vi "Module Top Level.vi"(8 "error in (no error)":errorcluster) -> (0 "error out":errorcluster)   [LabVIEW 2018, in "Controller (Host).lvlib"]
doc: "This is the top level VI for this module. It uses a queue for communications and is stopped using a user event. The general architecture is similar to a simple queued message handler.\n\nThis module controls the host computer logic, specifically the following:\nSplash screen deployment for user selections (APU selection, Operation selection)\nUser Interface visual deployment during operation"
uses:
  Controller (Host).lvlib
  Private Controls/Controller (Host) Data.ctl
  Private Controls/State.ctl
  Top Level/Shared Controls/APU Setup File.ctl
  Public Controls/Test Information.ctl
  Public VIs/PreorPostSB.ctl
  Public Controls/APU Select.ctl
  Top Level/Shared Controls/Calculated Data.ctl
  Private Controls/Module Data.ctl
  Private Controls/Module Action.ctl
  Top Level/Shared Controls/All Data Cluster.ctl
  Top Level/Shared Controls/Acq Data.ctl
  Globals/Host Globals.vi
  Error Handler/Error Handler.lvlib
  File IO/File IO.lvlib
  Testing UI 1/Testing UI 1.lvlib
  Testing UI 3/Testing UI 3.lvlib
  Testing UI 2/Testing UI 2.lvlib
  Fuel Farm/Fuel Farm.lvlib
panel:
  # "CONTROLLER"
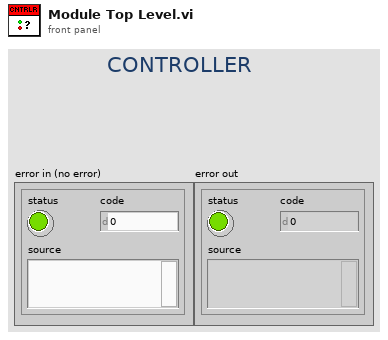
[diagram p1: front panel]
types:
  T1 = typedef "Controller (Host).lvlib/Controller (Host) Data.ctl" = cluster{"State":T2, "2D User Info":string[][], "APU Setup File":T3, "Test Information":T4, "ChannelTags":string[], "Live_Min_Max_Dev":dbl[][], "CalChannels":string[], "Slopes":dbl[], "Offsets":dbl[], "Calculated Values":T7, "ThresholdChannels":string[], "ThresholdRPM":dbl[], "ThresholdMin":bool[], "ThresholdValue":dbl[], "HeavyCCM":dbl[][], "LightCCM":dbl[][], "FuelFarm":bool}
  T2 = typedef "Controller (Host).lvlib/State.ctl" = enum16{"APU Select", "Operation Select", "SubTests Select", "Calibration", "Testing", "Exit"}
  T3 = typedef "APU Setup File.ctl" = cluster{"Sensor Info":string[][], "Variables":string[][], "CMM Table 106":string[][], "CMM Table 106B ":string[][], "Accel Config":string[][], "Report Sheet 1":string[][], "Report Sheet 2":string[][], "Report Sheet 3":string[][]}
  T4 = typedef "Controller (Host).lvlib/Test Information.ctl" = cluster{"APU Part Number:":string, "Model:":string, "Serial Number:":string, "Customer:":string, "Work Order:":string, "Pre or Post SB":T5, "Run Count":i32, "APU Selected":T6}
  T5 = typedef "Controller (Host).lvlib/PreorPostSB.ctl" = string
  T6 = typedef "Controller (Host).lvlib/APU Select.ctl" = string
  T7 = typedef "Calculated Data.ctl" = cluster{"C.00":dbl, "C.01":dbl, "C.02":dbl, "C.03":dbl, "C.04":dbl, "C.05":dbl, "C.06":dbl, "C.07":dbl, "C.08":dbl, "C.09":dbl, "C.10":dbl, "C.11":dbl, "C.12":dbl, "C.13":dbl, "C.14":dbl, "C.15":dbl, "C.16":dbl, "C.17":dbl, "C.18":dbl, "C.19":dbl, "C.20":dbl, "C.21":dbl, "C.22":dbl, "C.23":dbl, "C.24":dbl, "C.25":dbl, "C.26":dbl, "C.27":dbl, "C.28":dbl, "C.29":dbl, "C.30":dbl, "C.31":dbl, "C.32":dbl, "C.33":dbl, "C.34":dbl, "C.35":dbl, "C.36":dbl, "C.37":dbl, "C.38":dbl, "C.39":dbl, "C.40":dbl, "C.41":dbl, "C.42":dbl, "C.43":dbl, "C.44":dbl, "C.45":dbl, "C.46":dbl, "C.47":dbl, "C.48":dbl, "C.49":dbl, "C.50":dbl, "C.51":dbl, "C.52":dbl, "C.53":dbl, "C.54":dbl, "C.55":dbl, "C.56":dbl, "C.57":dbl, "C.58":dbl, "C.59":dbl, "C.60":dbl, "C.61":dbl, "C.62":dbl}
  T8 = typedef "All Data Cluster.ctl" = cluster{"AI":T9, "Accel Data":cluster{"Accel RMS(in/sec2)":dbl[], "Accel Peak(in/sec2)":dbl[], "Velocity RMS(in/sec)":dbl[], "Velocity Peak(in/sec)":dbl[]}, "Temps":cluster{"01-00-9213":dbl[], "01-01-9213":dbl[], "01-02-9213":dbl[]}, "00-03-9402(RPM)":dbl[], "02-04-9871":dbl[], "ARINC":sgl[]}
  T9 = typedef "Acq Data.ctl" = cluster{"00-00-9220":dbl[], "00-01-9220":dbl[], "02-02-9219":dbl[], "02-03-9227":dbl[], "02-05-9205":dbl[]}
  T10 = typedef "Controller (Host).lvlib/Module Data.ctl" = cluster{"Data":variant, "Action":T11}
  T11 = typedef "Controller (Host).lvlib/Module Action.ctl" = enum8{"Timeout", "New Data", "Value to Monitor", "Init", "Reset Dev_Min_Max", "Error", "Exit", "Prompt Test Info", "Update Test Info", "Prompt Variable Info", "Load APU Setup Data"}
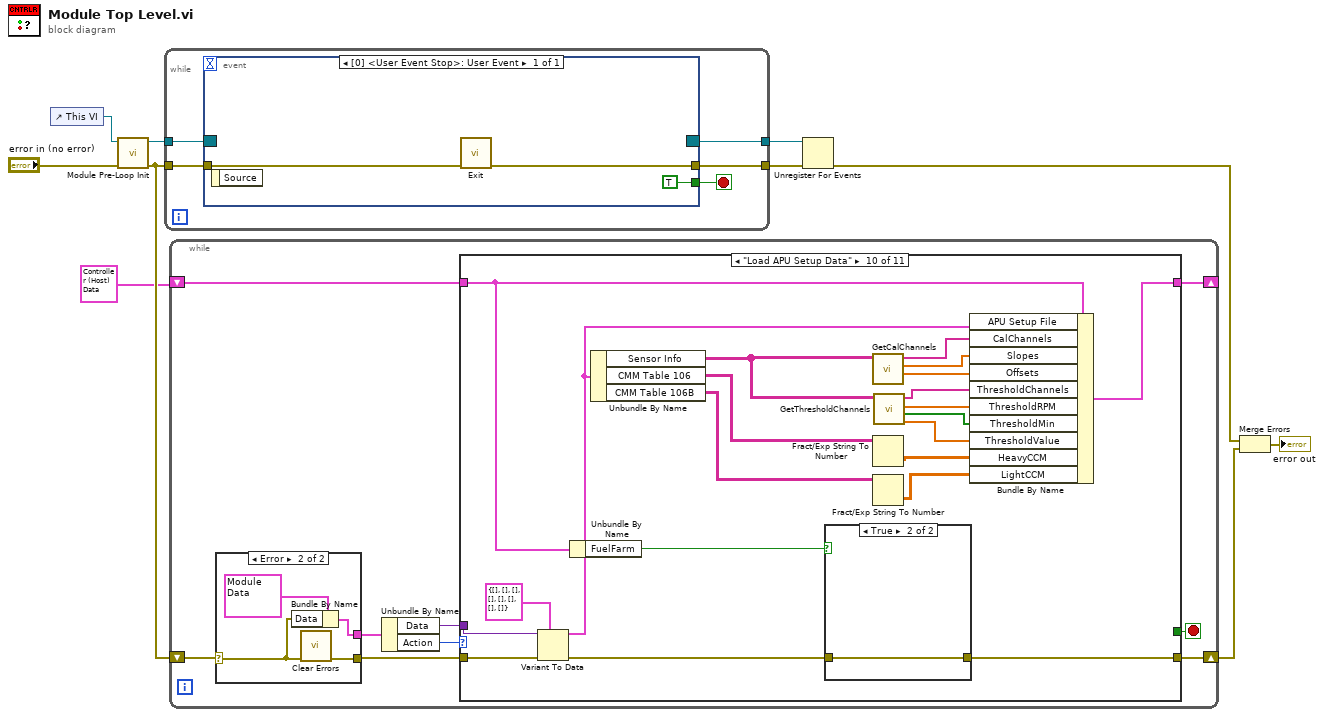
[diagram p0: block diagram]
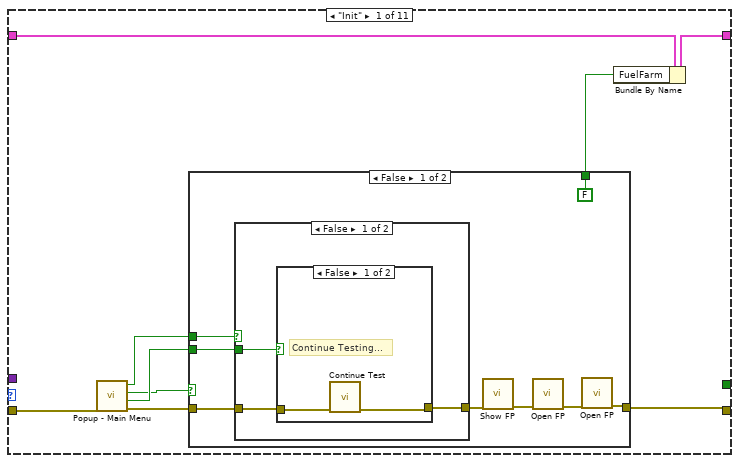
[diagram p2: hidden frame]
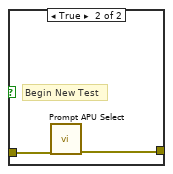
[diagram p3: hidden frame]
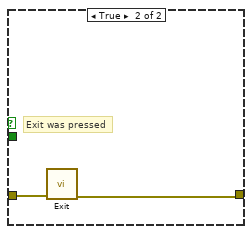
[diagram p4: hidden frame]
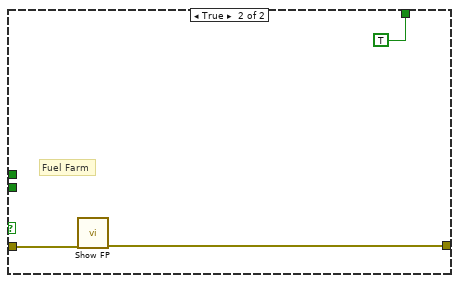
[diagram p5: hidden frame]
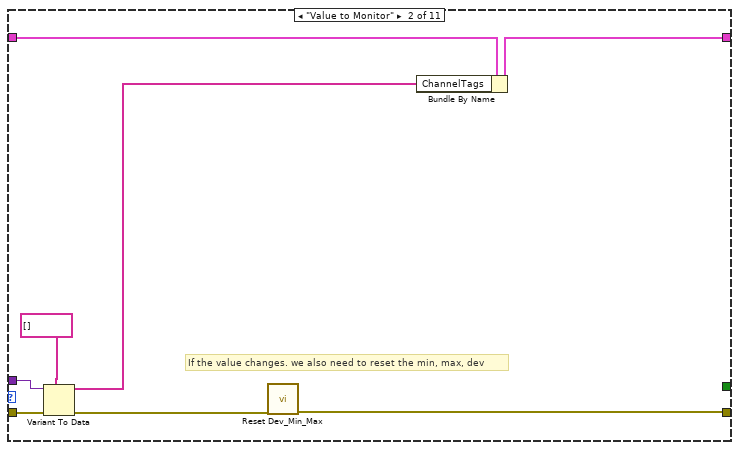
[diagram p6: hidden frame]
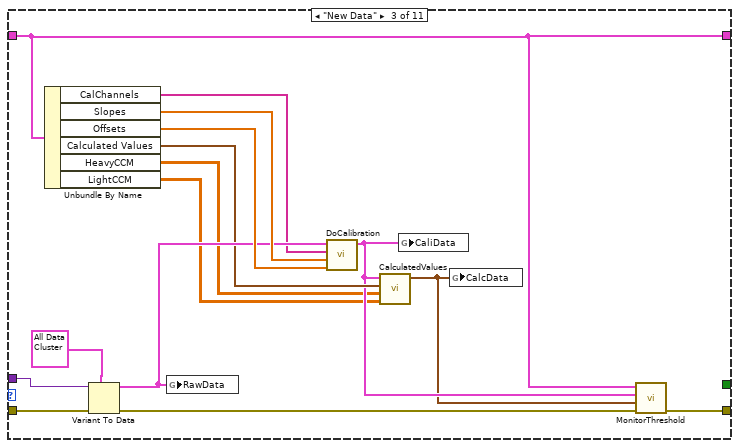
[diagram p7: hidden frame]
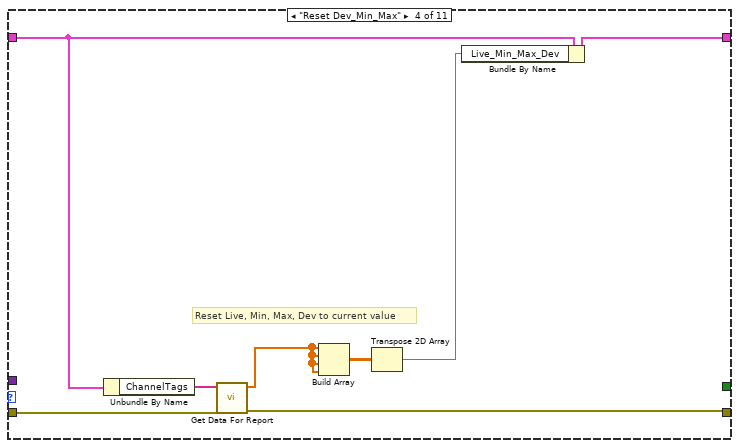
[diagram p8: hidden frame]
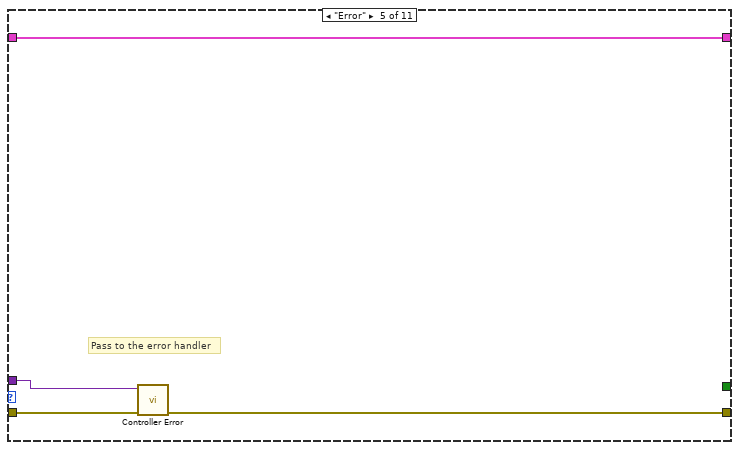
[diagram p9: hidden frame]
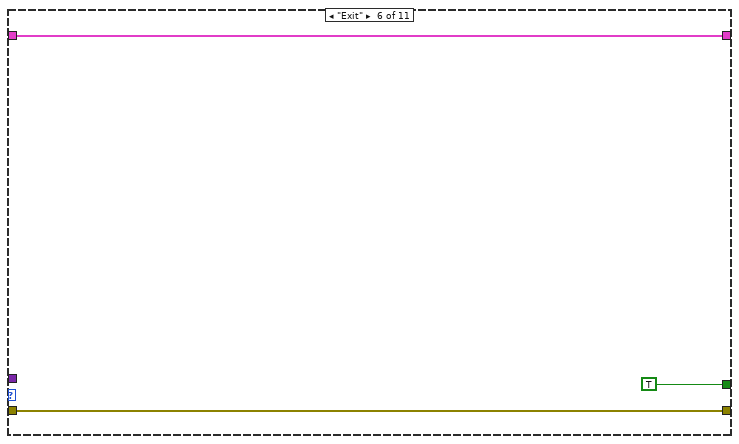
[diagram p10: hidden frame]
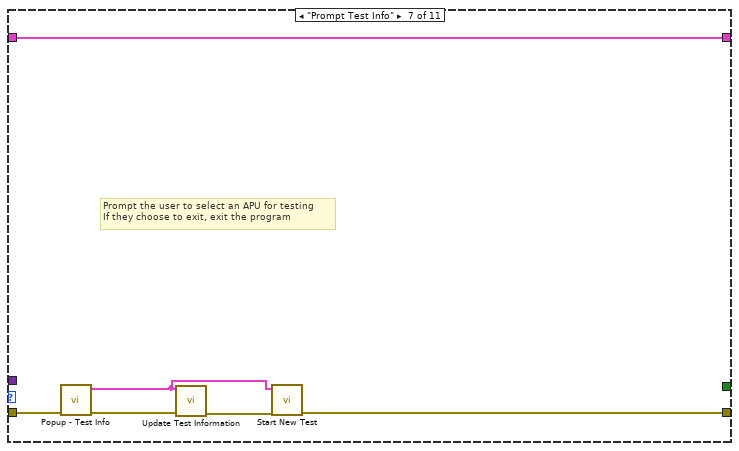
[diagram p11: hidden frame]
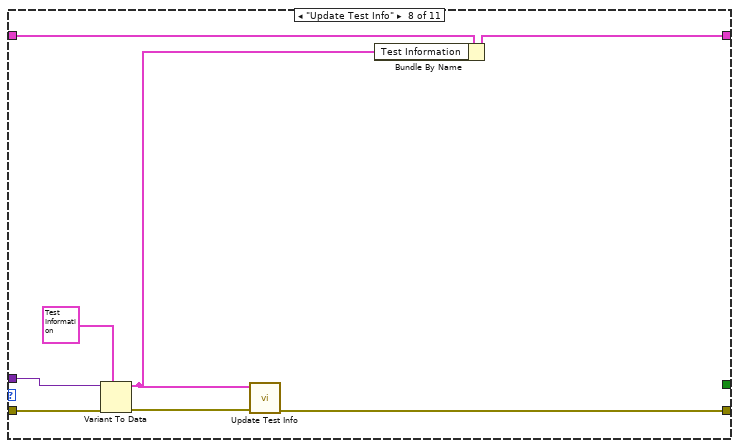
[diagram p12: hidden frame]
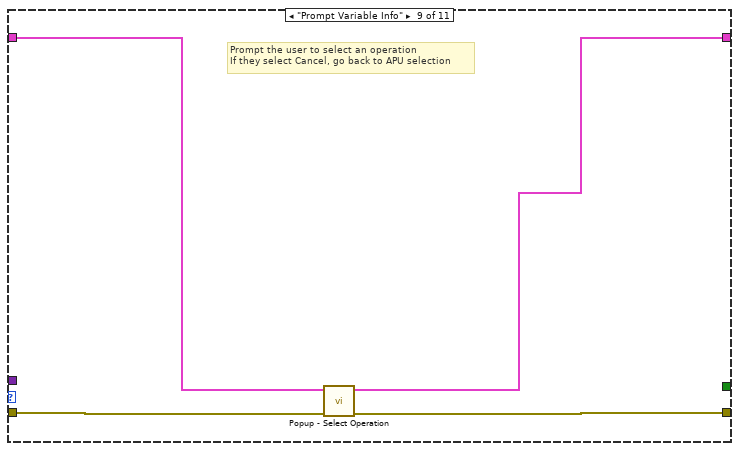
[diagram p13: hidden frame]
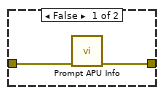
[diagram p14: hidden frame]
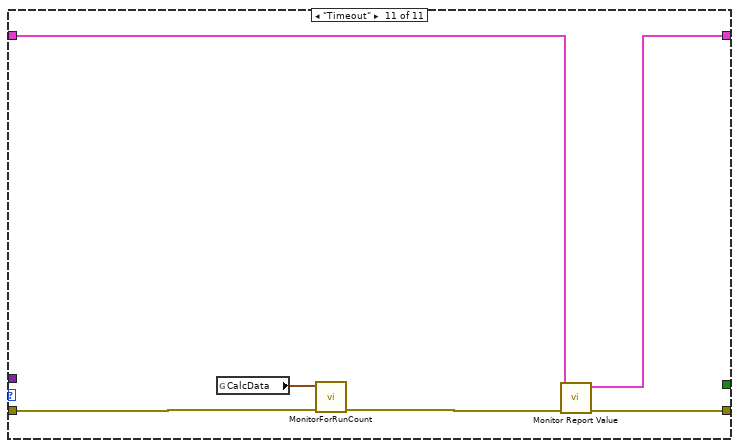
[diagram p15: hidden frame]
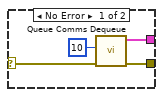
[diagram p16: hidden frame]
diagram:
  n1 = control-ref of="This VI"() -> (w10:refnum<vi>)
  n2 = call "Module Pre-Loop Init.vi"("error in (no error)"="error in (no error)", "Top Level VI Ref in"=w10) -> ("error out"=w2:errorcluster, "User Event Stop Ref"=w8:refnum<event-registration>)  [unwired: 8 in]
  n3 = while {
    tunnel: w8 -> [w15]
    tunnel: [w14] -> w6
    tunnel: w2 -> [w13]
    tunnel: [w11] -> w7
    stop <- w12 stop-if-true
    n4 = event shown="[0] <User Event Stop>: User Event" {
      selector: w15 -> [_]
      dyn-events: [_] -> w11
      timeout: _ -> [_]
      tunnel: [w16] -> w14
      tunnel: w13 -> [w17]
      tunnel: [TRUE] -> w12
      event User Event {
        n5 = event-data() -> ()  [unwired: 1 in, 1 out]
        n6 = call "Exit.vi"("error in"=w17) -> ("error out"=w16:errorcluster)  [unwired: 10 in]
      }
    }
  }
  n7 = while {
    shift-right: [w23] -> w5
    shift-left: w2 -> [w22]
    shift-right: [w21] -> _
    shift-left: T1 {"State"=enum."APU Select", "2D User Info"=[], "APU Setup File"={"Sensor Info"=[], "Variables"=[], "CMM Table 106"=[], "CMM Table 106B "=[], "Accel Config"=[], "Report Sheet 1"=[], "Report Sheet 2"=[], "Report Sheet 3"=[]}, "Test Information"={"APU Part Number:"="", "Model:"="", "Serial Number:"="", "Customer:"="", "Work Order:"="", "Pre or Post SB"="", "Run Count"=0, "APU Selected"="<Select>"}, "ChannelTags"=[], "Live_Min_Max_Dev"=[], "CalChannels"=[], "Slopes"=[], "Offsets"=[], "Calculated Values"={"C.00"=0.0, "C.01"=0.0, "C.02"=0.0, "C.03"=0.0, "C.04"=0.0, "C.05"=0.0, "C.06"=0.0, "C.07"=0.0, "C.08"=0.0, "C.09"=0.0, "C.10"=0.0, "C.11"=0.0, "C.12"=0.0, "C.13"=0.0, "C.14"=0.0, "C.15"=0.0, "C.16"=0.0, "C.17"=0.0, "C.18"=0.0, "C.19"=0.0, "C.20"=0.0, "C.21"=0.0, "C.22"=0.0, "C.23"=0.0, "C.24"=0.0, "C.25"=0.0, "C.26"=0.0, "C.27"=0.0, "C.28"=0.0, "C.29"=0.0, "C.30"=0.0, "C.31"=0.0, "C.32"=0.0, "C.33"=0.0, "C.34"=0.0, "C.35"=0.0, "C.36"=0.0, "C.37"=0.0, "C.38"=0.0, "C.39"=0.0, "C.40"=0.0, "C.41"=0.0, "C.42"=0.0, "C.43"=0.0, "C.44"=0.0, "C.45"=0.0, "C.46"=0.0, "C.47"=0.0, "C.48"=0.0, "C.49"=0.0, "C.50"=0.0, "C.51"=0.0, "C.52"=0.0, "C.53"=0.0, "C.54"=0.0, "C.55"=0.0, "C.56"=0.0, "C.57"=0.0, "C.58"=0.0, "C.59"=0.0, "C.60"=0.0, "C.61"=0.0, "C.62"=0.0}, "ThresholdChannels"=[], "ThresholdRPM"=[], "ThresholdMin"=[], "ThresholdValue"=[], "HeavyCCM"=[], "LightCCM"=[], "FuelFarm"=FALSE} -> [w20]
    stop <- w24 stop-if-true
    n8 = case shown="Error" w22 {
      selector: w22 -> [w145 w148]
      tunnel: [w146 w149] -> w27
      tunnel: [w144 w147] -> w25
      frame No Error {
        n9 = call "Queue Comms Dequeue.vi"("error in (no error)"=w145, "timeout in ms (-1)"=10) -> ("error out"=w144:errorcluster, "element"=w146:T10)  [unwired: 8 in]
      }
      frame Error {
        n10 = Bundle By Name(cluster=T10 {"Data"=variant, "Action"=enum."Error"} ("element"), "Data"=w148) -> (w149:T10)
        n11 = call <vilib>:"Clear Errors.vi"("error in (no error)"=w148) -> ("error out"=w147:errorcluster)  [unwired: 5 in, 1 out]
      }
    }
    n12 = Unbundle By Name(w27) -> ("Data"=w26:variant, "Action"=w19:T11)
    n13 = case shown="\"Load APU Setup Data\"" w19 {
      tunnel: w26 -> [_ w61 w78 _ w89 _ _ w106 _ w133 _]
      tunnel: w25 -> [w35 w63 w79 w87 w91 w93 w99 w107 w112 w132 w142]
      tunnel: [w36 w57 w68 w83 w90 w93 w96 w102 w111 w129 w140] -> w23
      tunnel: [_ _ _ _ _ TRUE _ _ _ _ _] -> w24
      tunnel: [w29 w60 w67 w84 w88 w92 w100 w104 w110 w127 w139] -> w21
      tunnel: w20 -> [w30 w64 w67 w86 w88 w92 w100 w108 w109 w114 w138]
      frame "Init" {
        n14 = call "Popup - Main Menu.vi"("error in"=w35) -> ("error out"=w34:errorcluster, "IsNewTest"=w33:bool, "FuelFarm"=w31:bool, "Exit"=w32:bool)  [unwired: 7 in]
        n15 = case shown="False" w31 {
          tunnel: [w38 w55] -> w36
          tunnel: w34 -> [w44 w56]
          tunnel: w33 -> [w43 _]
          tunnel: w32 -> [w42 _]
          tunnel: [FALSE TRUE] -> w28
          frame False {
            n16 = case shown="False" w42 {
              tunnel: [w47 w52] -> w41
              tunnel: w44 -> [w46 w53]
              tunnel: w43 -> [w45 _]
              frame False {
                n17 = case shown="False" w45 {
                  tunnel: w46 -> [w49 w51]
                  tunnel: [w48 w50] -> w47
                  frame False {
                    # "Continue Testing..."
                    n18 = call "Continue Test.vi"("error in (no error)"=w49) -> ("error out"=w48:errorcluster)  [unwired: 10 in]
                  }
                  frame True {
                    # "Begin New Test"
                    n19 = call "Prompt APU Select.vi"("error in (no error)"=w51) -> ("error out"=w50:errorcluster)  [unwired: 10 in]
                  }
                }
              }
              frame True {
                # "Exit was pressed"
                n20 = call "Exit.vi"("error in"=w53) -> ("error out"=w52:errorcluster)  [unwired: 10 in]
              }
            }
            n21 = call "Show FP.vi"("error in (no error)"=w41) -> ("error out"=w40:errorcluster)  [unwired: 10 in]
            n22 = call "Open FP.vi"("error in (no error)"=w40) -> ("error out"=w39:errorcluster)  [unwired: 10 in]
            n23 = call "Open FP.vi"("error in (no error)"=w39) -> ("error out"=w38:errorcluster)  [unwired: 10 in]
          }
          frame True {
            # "Fuel Farm"
            n24 = call "Show FP.vi"("error in (no error)"=w56) -> ("error out"=w55:errorcluster)  [unwired: 10 in]
          }
        }
        n25 = Bundle By Name(cluster=w30, "FuelFarm"=w28) -> (w29:T1)
      }
      frame "Value to Monitor" {
        # "If the value changes. we also need to reset the min, max, dev"
        n26 = Variant To Data(error in=w63, type=string[] [], Variant=w61) -> (data=w59:string[], error out=w58:errorcluster)
        n27 = call "Reset Dev_Min_Max.vi"("error in (no error)"=w58) -> ("error out"=w57:errorcluster)  [unwired: 10 in]
        n28 = Bundle By Name(cluster=w64, "ChannelTags"=w59) -> (w60:T1)
      }
      frame "New Data" {
        n29 = Unbundle By Name(w67) -> ("CalChannels"=w72:string[], "Slopes"=w76:dbl[], "Offsets"=w75:dbl[], "Calculated Values"=w73:T7, "HeavyCCM"=w66:dbl[][], "LightCCM"=w65:dbl[][])
        n30 = Variant To Data(error in=w79, type=T8 {"AI"={"00-00-9220"=[], "00-01-9220"=[], "02-02-9219"=[], "02-03-9227"=[], "02-05-9205"=[]}, "Accel Data"={"Accel RMS(in/sec2)"=[], "Accel Peak(in/sec2)"=[], "Velocity RMS(in/sec)"=[], "Velocity Peak(in/sec)"=[]}, "Temps"={"01-00-9213"=[], "01-01-9213"=[], "01-02-9213"=[]}, "00-03-9402(RPM)"=[], "02-04-9871"=[], "ARINC"=[]} ("All Data Cluster"), Variant=w78) -> (data=w74:T8, error out=w69:errorcluster)
        n31 = global write "Host Globals.vi" "RawData"(w74) -> ()
        n32 = call "DoCalibration.vi"("Offsets"=w75, "Slopes"=w76, "Channel Tags"=w72, "Data"=w74) -> ("DataOut"=w71:T8)  [unwired: 7 in]
        n33 = call "CalculatedValues.vi"("CCM LM"=w65, "CCM H"=w66, "Calculated Values"=w73, "Data"=w71) -> ("Calculated Values"=w70:T7)  [unwired: 7 in]
        n34 = global write "Host Globals.vi" "CaliData"(w71) -> ()
        n35 = global write "Host Globals.vi" "CalcData"(w70) -> ()
        n36 = call "MonitorThreshold.vi"("error constant"=w69, "CalcData"=w70, "CaliData"=w71, "Data"=w67) -> ("error out"=w68:errorcluster)  [unwired: 7 in]
      }
      frame "Reset Dev_Min_Max" {
        # "Reset Live, Min, Max, Dev to current value"
        n37 = Unbundle By Name(w86) -> ("ChannelTags"=w85:string[])
        n38 = call "Get Data For Report.vi"("error constant"=w87, "Channel Tags"=w85) -> ("error out"=w83:errorcluster, "Value"=w82:dbl[])  [unwired: 8 in]
        n39 = Build Array(w82, w82, w82, w82) -> (w81:dbl[][])
        n40 = Transpose 2D Array(2D array=w81) -> (transposed array=w80:dbl[][])
        n41 = Bundle By Name(cluster=w86, "Live_Min_Max_Dev"=w80) -> (w84:T1)
      }
      frame "Error" {
        # "Pass to the error handler"
        n42 = call "Controller Error.vi"("error in (no error)"=w91, "Data"=w89) -> ("error out"=w90:errorcluster)  [unwired: 9 in]
      }
      frame "Exit" {
      }
      frame "Prompt Test Info" {
        # "Prompt the user to select an APU for testing\nIf they choose to exit, exit the program"
        n43 = call "Popup - Test Info.vi"("error i"=w99) -> ("error out"=w98:errorcluster, "Test Information out"=w95:T4)  [unwired: 9 in]
        n44 = call "Update Test Information.vi"("error in"=w98, "Test Information"=w95) -> ("error out"=w97:errorcluster)  [unwired: 9 in]
        n45 = call "Start New Test.vi"("error in (no error)"=w97, "Test Information"=w95) -> ("error out"=w96:errorcluster)  [unwired: 9 in]
      }
      frame "Update Test Info" {
        n46 = Variant To Data(error in=w107, type=T4 {"APU Part Number:"="555", "Model:"="5", "Serial Number:"="sad", "Customer:"="sad", "Work Order:"="asd", "Pre or Post SB"="Pre SB 49-7711", "Run Count"=0, "APU Selected"="<Select>"} ("Test Information"), Variant=w106) -> (data=w103:T4, error out=w101:errorcluster)
        n47 = call "Update Test Info.vi"("error in (no error)"=w101, "Test Information"=w103) -> ("error out"=w102:errorcluster)  [unwired: 9 in]
        n48 = Bundle By Name(cluster=w108, "Test Information"=w103) -> (w104:T1)
      }
      frame "Prompt Variable Info" {
        # "Prompt the user to select an operation\nIf they select Cancel, go back to APU selection"
        n49 = call "Popup - Select Operation.vi"("error in (no error)"=w112, "Controller (Host) Data in"=w109) -> ("error out"=w111:errorcluster, "Controller (Host) Data out"=w110:T1)  [unwired: 8 in]
      }
      frame "Load APU Setup Data" {
        n50 = Variant To Data(error in=w132, type=T3 {"Sensor Info"=[], "Variables"=[], "CMM Table 106"=[], "CMM Table 106B "=[], "Accel Config"=[], "Report Sheet 1"=[], "Report Sheet 2"=[], "Report Sheet 3"=[]} ("APU Setup File"), Variant=w133) -> (data=w128:T3, error out=w130:errorcluster)
        n51 = Unbundle By Name(w114) -> ("FuelFarm"=w113:bool)
        n52 = Unbundle By Name(w128) -> ("Sensor Info"=w123:string[][], "CMM Table 106"=w118:string[][], "CMM Table 106B"=w116:string[][])
        n53 = case shown="True" w113 {
          tunnel: w130 -> [w135 w136]
          tunnel: [w134 w136] -> w129
          frame False {
            n54 = call "Prompt APU Info.vi"("error in (no error)"=w135) -> ("error out"=w134:errorcluster)  [unwired: 10 in]
          }
          frame True {
          }
        }
        n55 = call "GetCalChannels.vi"("Sensor Info"=w123) -> ("Offsets"=w124:dbl[], "Slopes"=w125:dbl[], "CalChannels"=w126:string[])  [unwired: 8 in]
        n56 = Fract/Exp String To Number(string=w118) -> (number=w117:dbl[][])  [unwired: 3 in, 1 out]
        n57 = Fract/Exp String To Number(string=w116) -> (number=w115:dbl[][])  [unwired: 3 in, 1 out]
        n58 = call "GetThresholdChannels.vi"("Sensor Info"=w123) -> ("ThresholdValue"=w119:dbl[], "IsMinThreshold"=w120:bool[], "RPM Engage"=w121:dbl[], "ThresholdChannels"=w122:string[])  [unwired: 7 in]
        n59 = Bundle By Name(cluster=w114, "APU Setup File"=w128, "CalChannels"=w126, "Slopes"=w125, "Offsets"=w124, "ThresholdChannels"=w122, "ThresholdRPM"=w121, "ThresholdMin"=w120, "ThresholdValue"=w119, "HeavyCCM"=w117, "LightCCM"=w115) -> (w127:T1)
      }
      frame "Timeout" {
        n60 = global read "Host Globals.vi" "CalcData"() -> (w137:T7)
        n61 = call "MonitorForRunCount.vi"("error in (no error)"=w142, "Calculated Values"=w137) -> ("error out"=w141:errorcluster)  [unwired: 9 in]
        n62 = call "Monitor Report Value.vi"("error in"=w141, "DataIn"=w138) -> ("error out"=w140:errorcluster, "DataOut"=w139:T1)  [unwired: 8 in]
      }
    }
  }
  n63 = Unregister For Events(event registration refnum=w7, error in=w6) -> (error out=w3:errorcluster)
  n64 = Merge Errors(w3, w5) -> (→"error out":errorcluster)
